vi "MCA Tank Controller Local HMI (Debug).vi"() -> ()   [LabVIEW 2013]
uses:
  <vilib>/NI/Current Value Table/Write.vi
  <vilib>/NI/Current Value Table/DataTypes/Boolean_Write.vi
  <vilib>/NI/Current Value Table/Static Read.vi
  <vilib>/NI/Current Value Table/DataTypes/Double_Static Read.vi
  <vilib>/NI/Current Value Table/DataTypes/Boolean_Static Read.vi
  <vilib>/NI/Current Value Table/Type to Enum.vi
  <vilib>/NI/Current Value Table/DataTypes/Boolean_Type To Enum.vi
  <vilib>/NI/Current Value Table/DataTypes/Double_Type To Enum.vi
  <vilib>/NI/Current Value Table/FGVs/CVT Globals.vi
  <vilib>/NI/Current Value Table/FGVs/Tag Memory.vi
  <vilib>/NI/Current Value Table/Memory Block.vi
  <vilib>/NI/Current Value Table/DataTypes/Boolean_Memory Block.vi
  <vilib>/NI/Current Value Table/DataTypes/Double_Memory Block.vi
panel:
  in  "stop":bool
  in  "Tab Control":T1(tab)
  out "Drain Valve":bool
  in  "Start":bool
  out "Temperature":dbl(slide) scale=0.0..10.0
  out "Fill Valve":bool
  out "Heater":bool
  out "Tank":dbl(slide) scale=0.0..10.0
  out "Timer":dbl format="%.2g"
  in  "Enable":bool
  in  "Heater":bool
  in  "Drain Valve":bool
  in  "Fill Valve":bool
  out "Heater":bool
  out "Drain Valve":bool
  out "Fill Valve":bool
  out "Fill Level":dbl
  out "Temperature":dbl
  # "Tank Control Debug HMI"
  # "Process Logic:\n- Fill Tank to level >= 5\n- Heat Tank to\n  Temperature>= 5\n- Wait 5 seconds\n- Drain Tank"
  # "CVT Values"
  # "Manual Control"
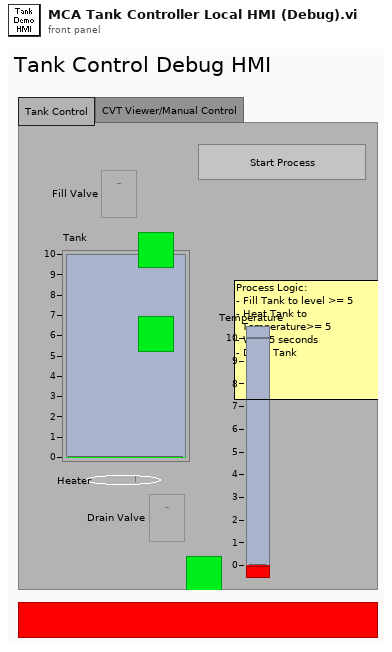
[diagram p1: front panel]
types:
  T1 = enum32{"Tank Control", "CVT Viewer/Manual Control"}
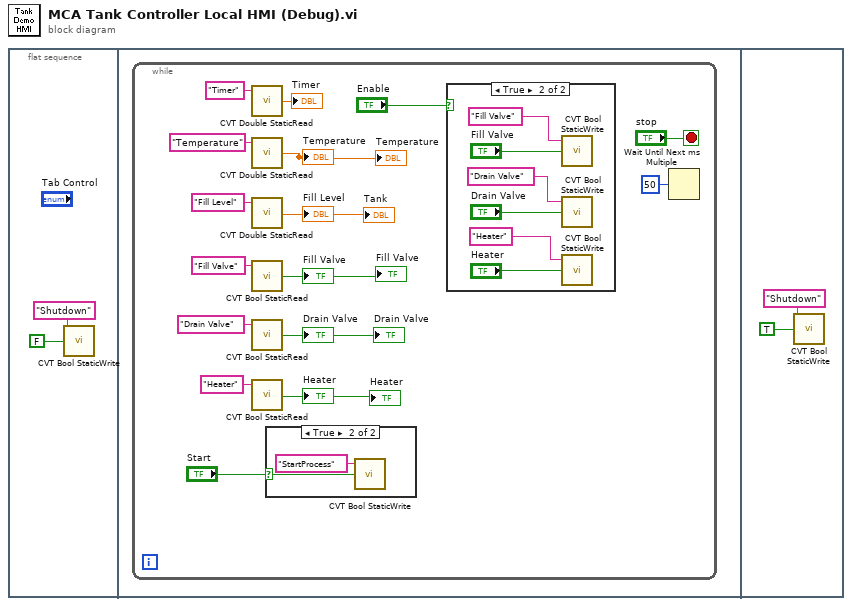
[diagram p0: block diagram]
diagram:
  n1 = flat-sequence {
    frame #0 {
      n2 = call <vilib>:"CVT Bool StaticWrite.vi"("Value"=FALSE, "Tag Name"="Shutdown") -> ()  [unwired: 3 in, 1 out]
    }
    frame #1 {
      n3 = while {
        stop <- "stop" stop-if-true
        n4 = call <vilib>:"CVT Double StaticRead.vi"("Tag Name"="Timer") -> ("Value"=→"Timer":dbl)  [unwired: 3 in, 1 out]
        n5 = call <vilib>:"CVT Double StaticRead.vi"("Tag Name"="Temperature") -> ("Value"=→"Temperature" →"Temperature":dbl)  [unwired: 3 in, 1 out]
        n6 = call <vilib>:"CVT Double StaticRead.vi"("Tag Name"="Fill Level") -> ("Value"=→"Fill Level" →"Tank":dbl)  [unwired: 3 in, 1 out]
        n7 = call <vilib>:"CVT Bool StaticRead.vi"("Tag Name"="Fill Valve") -> ("Value"=→"Fill Valve" →"Fill Valve":bool)  [unwired: 3 in, 1 out]
        n8 = call <vilib>:"CVT Bool StaticRead.vi"("Tag Name"="Drain Valve") -> ("Value"=→"Drain Valve" →"Drain Valve":bool)  [unwired: 3 in, 1 out]
        n9 = call <vilib>:"CVT Bool StaticRead.vi"("Tag Name"="Heater") -> ("Value"=→"Heater" →"Heater":bool)  [unwired: 3 in, 1 out]
        n10 = case shown="True" "Start" {
          selector: "Start" -> [_ w19]
          frame False {
          }
          frame True {
            n11 = call <vilib>:"CVT Bool StaticWrite.vi"("Value"=w19, "Tag Name"="StartProcess") -> ()  [unwired: 3 in, 1 out]
          }
        }
        n12 = case shown="True" "Enable" {
          frame False {
          }
          frame True {
            n13 = call <vilib>:"CVT Bool StaticWrite.vi"("Value"="Fill Valve", "Tag Name"="Fill Valve") -> ()  [unwired: 3 in, 1 out]
            n14 = call <vilib>:"CVT Bool StaticWrite.vi"("Value"="Drain Valve", "Tag Name"="Drain Valve") -> ()  [unwired: 3 in, 1 out]
            n15 = call <vilib>:"CVT Bool StaticWrite.vi"("Value"="Heater", "Tag Name"="Heater") -> ()  [unwired: 3 in, 1 out]
          }
        }
        n16 = Wait Until Next ms Multiple(millisecond multiple=u32 50) -> ()  [unwired: 1 out]
      }
    }
    frame #2 {
      n17 = call <vilib>:"CVT Bool StaticWrite.vi"("Value"=TRUE, "Tag Name"="Shutdown") -> ()  [unwired: 3 in, 1 out]
    }
  }
